vi "(SubVI)Init GV.vi"(8 "error in (no error)":errorcluster caption="에러 입력(에러 없음)") -> (0 "error out":errorcluster caption="에러 출력")   [LabVIEW 2020]
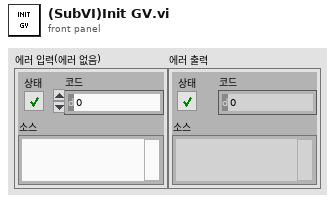
[diagram p1: front panel]
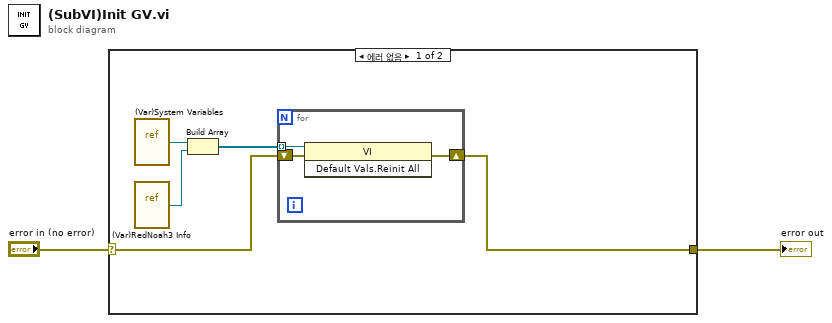
[diagram p0: block diagram]
diagram:
  n1 = case shown="에러 없음" "error in (no error)" {
    selector: "error in (no error)" -> [w6 w11]
    tunnel: [w5 w11] -> w1
    frame No Error {
      n2 = vi-ref "(Var)System Variables.vi"() -> (w7:refnum<vi>)
      n3 = vi-ref "(Var)RedNoah3 Info.vi"() -> (w3:refnum<vi>)
      n4 = Build Array(w7, w3) -> (w4:refnum<vi>[])
      n5 = for {
        tunnel: w4 -> [w10] mode=indexing
        shift-right: [w8] -> w5
        shift-left: w6 -> [w9]
        n6 = invoke class="VI" method="Default Vals.Reinit All"(reference=w10, error in=w9) -> (error out=w8:errorcluster)  [unwired: 1 in, 2 out]
      }
    }
    frame Error {
    }
  }
  "error out" <- w1
